vi "Gas_Release_Control.vi"(5 "Extra Commands":string, 6 "Density Ratio":string="Carrier 1 only", 7 "Strength (% by volume)":dbl format="%.3f", 8 "Stack flowrate (l/min)":dbl format="%.2f", 9 "Source Status":T2) -> (0 "error out":errorcluster, 1 "Flowrates (kg/min)":dbl[](array[numeric]) format="%.2f", 2 "Source Est Time (s)":dbl, 3 "Flowrates Achieved?":bool)   [LabVIEW 2011]
uses:
  ADAM Controls/Client_Source_Status.ctl
  ADAM Controls/Client_Source.ctl
  ADAM Controls/Channel_names.ctl
  ADAM Controls/Ch_description_ADAM.ctl
  ADAM Controls/Module_type_ADAM.ctl
  ADAM Controls/Function_ADAM.ctl
  ADAM Controls/Channel_State.ctl
  ADAM Controls/Calib_type_ADAM.ctl
  ADAM Controls/Address.ctl
  ADAM Controls/Update_scan_value.ctl
  Anemometry/Anemometry Sub Vis/Controls/In_Range.ctl
  Anemometry/Anemometry Sub Vis/Globals/Preference_global.vi
  Anemometry/Anemometry Sub Vis/Globals/Extra_Commands_Global.vi
panel:
  out "Error String":string
  out "Currently on":T1=enum."Get Source Clients"
  out "Status of other Clients":string[](array[string])
  out "Source already correct?":bool
  out "No Other Clients are Using Source?":bool
  out "Source Clients":string[](array[string])
  # "-Carrier 1 only\n-Carrier 2 only\n-Enter Ratio"
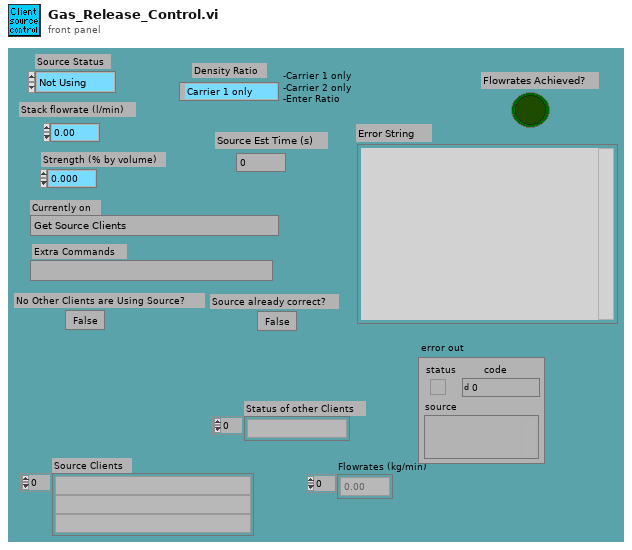
[diagram p1: front panel]
types:
  T1 = typedef "Client_Source.ctl" = enum16{"Start", "Get Source Clients", "Has this client liberty to control the source?", "Declare not using, other client already waiting", "Is the Source already correct?", "Declare waiting, other client is still using", "Control Hi-Tec", "Were the Hi-tecs able to achieve the flowrates?", "Declare source status", "Wait for source to Establish"}
  T2 = typedef "Client_Source_Status.ctl" = enum16{"Not Using", "Using", "Must Have"}
  T3 = typedef "Channel_names.ctl" = enum16{"Active Only", "Active + Off", "All Channels"}
  T4 = typedef "Ch_description_ADAM.ctl" = cluster{"Ch Name":string, "Type":T5, "Function":T6, "Ch State":T7, "Calibration type":T8, "A":dbl, "B":dbl, "C":dbl, "D":dbl, "Comments":string, "Address":T9, "String":string, "Duty":u16}
  T5 = typedef "Module_type_ADAM.ctl" = string
  T6 = typedef "Function_ADAM.ctl" = enum16{"Analogue Input", "Digital Input", "Event counter", "Event rate", "Analogue Output", "Digital Output", "Relay Output"}
  T7 = typedef "Channel_State.ctl" = enum16{"On", "Off", "Always On", "Always Off"}
  T8 = typedef "Calib_type_ADAM.ctl" = enum16{"Raw", "Bx + A", "Cx^2 + Bx + A", "Dx^3 + Cx^2 + Bx + A", "In Band", "Hi-Tec Q", "Hi-Tec M_dot", "Text"}
  T9 = typedef "Address.ctl" = cluster{"Main":i32, "Ch.":i32, "Sub":i32, "Port Name":string}
  T10 = typedef "Update_scan_value.ctl" = cluster{"Channel Name":string, "New Value":dbl}
  T11 = typedef "In_Range.ctl" = enum16{"%", "±", "% & ±"}
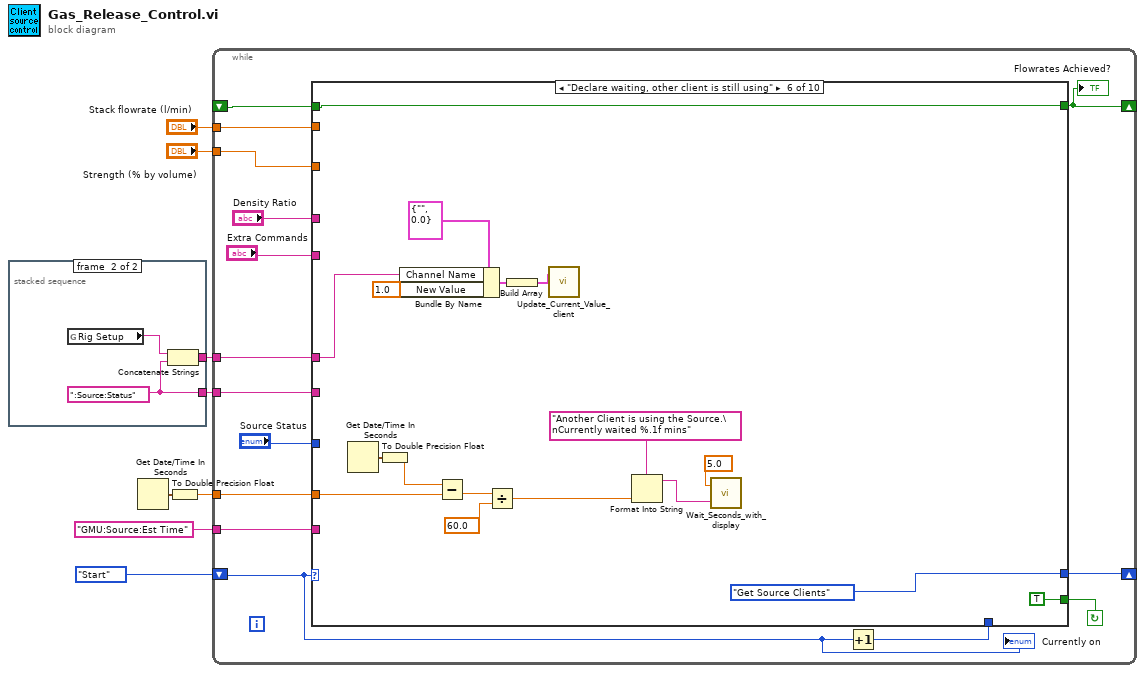
[diagram p0: block diagram]
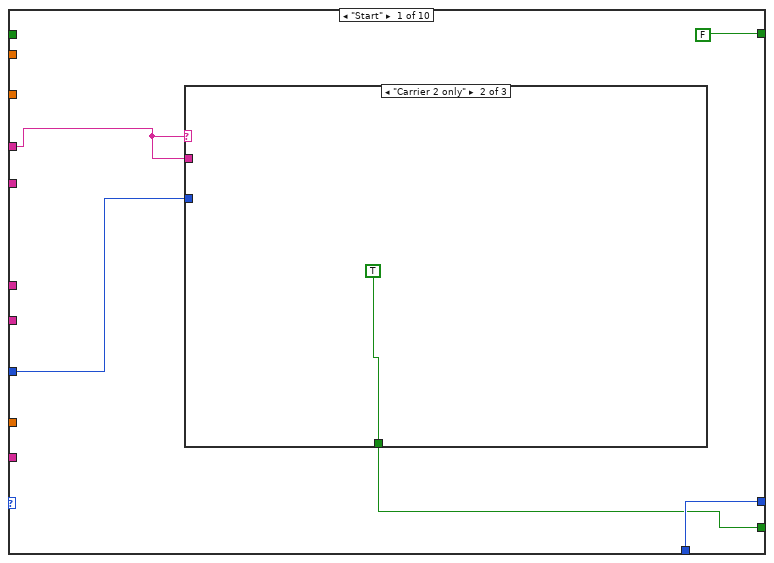
[diagram p2: hidden frame]
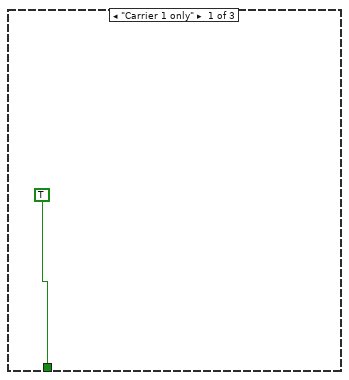
[diagram p3: hidden frame]
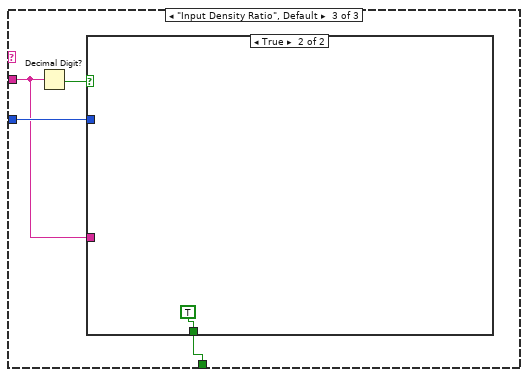
[diagram p4: hidden frame]
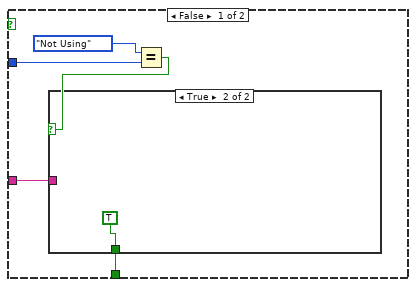
[diagram p5: hidden frame]
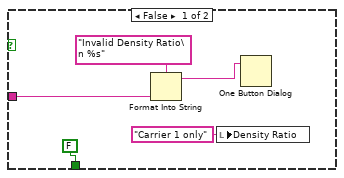
[diagram p6: hidden frame]
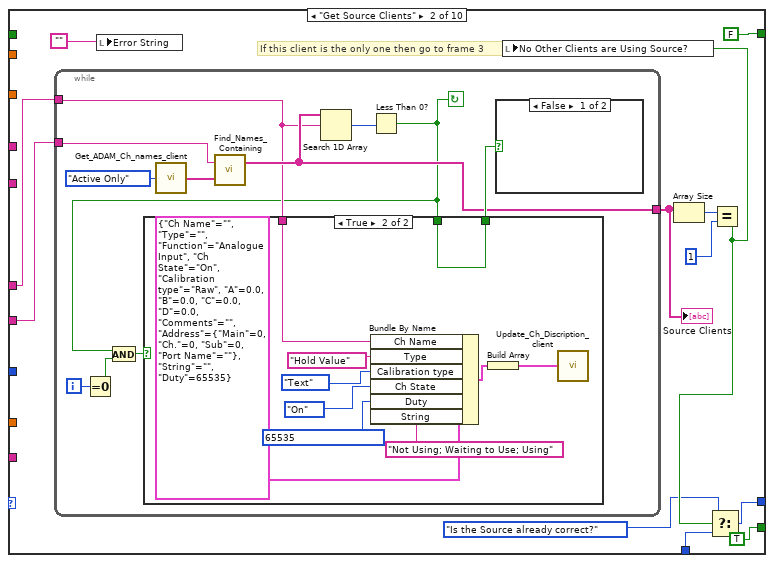
[diagram p7: hidden frame]
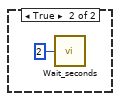
[diagram p8: hidden frame]
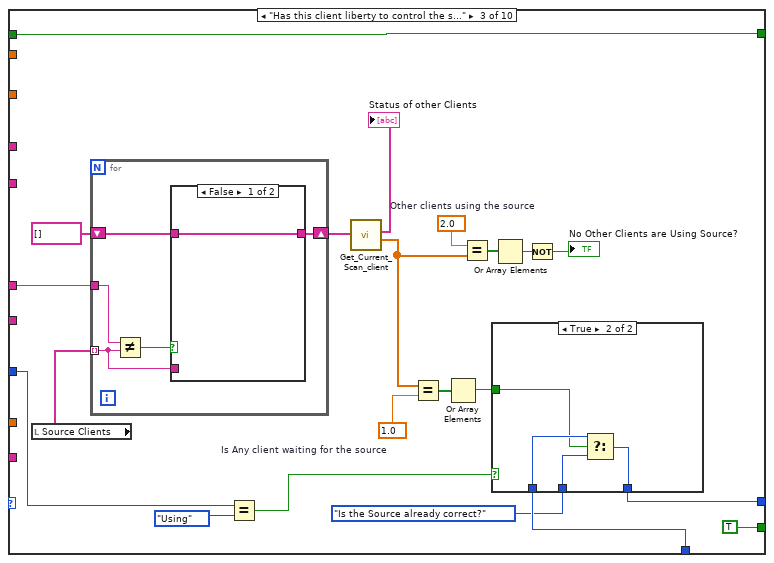
[diagram p10: hidden frame]
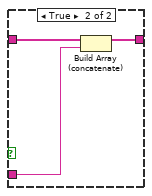
[diagram p12: hidden frame]
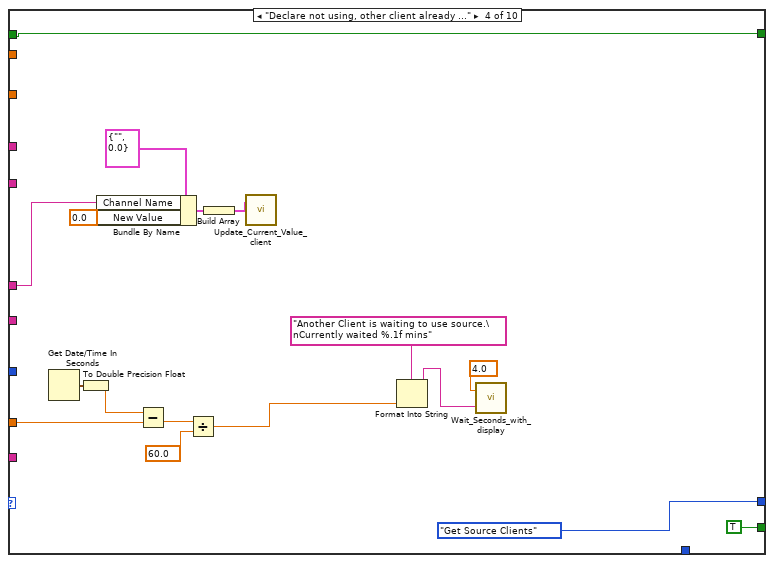
[diagram p13: hidden frame]
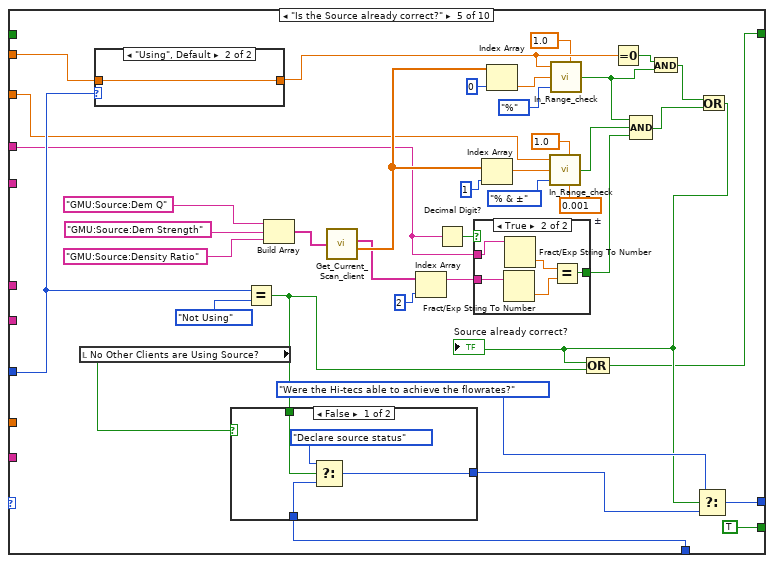
[diagram p14: hidden frame]
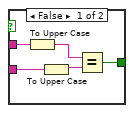
[diagram p15: hidden frame]
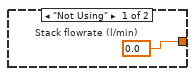
[diagram p16: hidden frame]
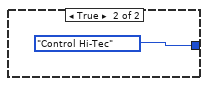
[diagram p17: hidden frame]
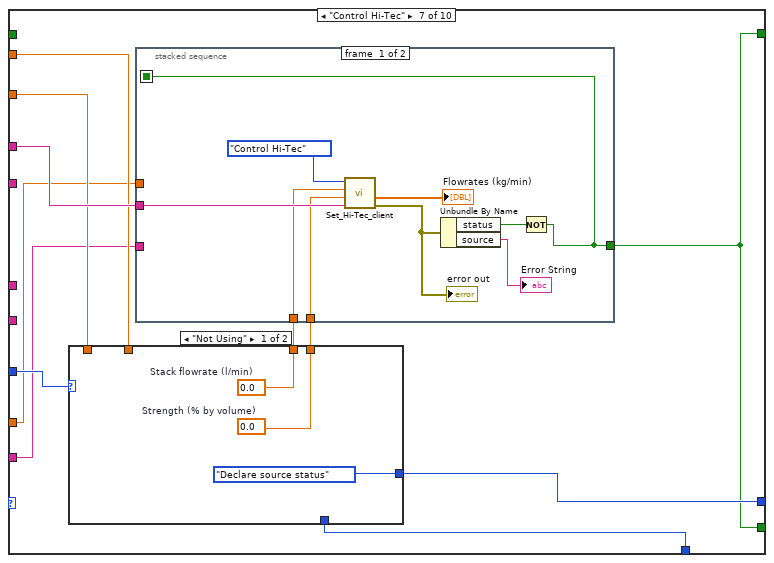
[diagram p18: hidden frame]
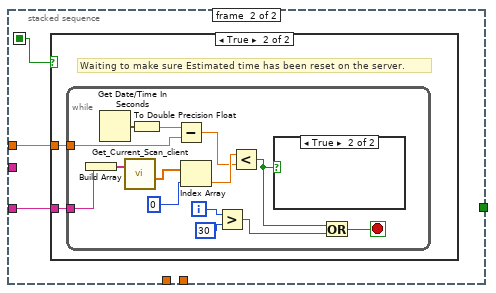
[diagram p19: hidden frame]
diagram:
  n1 = stacked-sequence {
    tunnel: [_ w11] -> w8
    tunnel: [_ w10] -> w7
    frame #0 {
      n2 = call "Run_EnFlo_Hub.vi"() -> ()  [unwired: 8 out]
    }
    frame #1 {
      w11 = ":Source:Status"
      n3 = global read "Preference_global.vi" "Rig Setup"() -> (w9:string)
      n4 = Concatenate Strings(w9, w11) -> (w10:string)
    }
  }
  n5 = Get Date/Time In Seconds() -> (seconds since 1Jan1904=w2:timestamp)
  n6 = To Double Precision Float(number=w2) -> (double precision float=w6:dbl)
  n7 = while {
    tunnel: w6 -> [w22]
    tunnel: w7 -> [w25]
    shift-left: Client_Source."Start" -> [w20]
    shift-right: [w21] -> _
    tunnel: w8 -> [w26]
    tunnel: "Stack flowrate (l/min)" -> [w16]
    tunnel: "Strength (% by volume)" -> [w15]
    shift-right: [w13] -> _
    shift-left: _ -> [w14]
    tunnel: "GMU:Source:Est Time" -> [w12]
    stop <- w24 continue-if-true
    n8 = Increment(x=w20) -> (x+1=w23:T1)
    n9 = case shown="\"Declare waiting, other client is still using\"" w20 {
      tunnel: w16 -> [_ _ _ _ w166 _ w217 w260 _ w308]
      tunnel: w15 -> [_ _ _ _ w147 _ w215 _ _ _]
      tunnel: "Density Ratio" -> [w30 _ _ _ w139 _ w220 _ _ _]
      tunnel: w26 -> [_ w61 _ _ _ _ _ _ _ _]
      tunnel: [w31 w57 w98 Client_Source."Get Source Clients" w175 Client_Source."Get Source Clients" w214 w262 w298 w314] -> w21
      tunnel: w25 -> [_ w60 w105 w131 _ w204 _ _ w304 _]
      tunnel: [w29 TRUE TRUE TRUE TRUE TRUE w210 TRUE TRUE FALSE] -> w24
      tunnel: w23 -> [w31 w56 w100 _ w167 _ w213 w261 w298 w314]
      tunnel: w22 -> [_ _ _ w129 _ w199 w211 _ _ _]
      tunnel: "Source Status" -> [w28 _ w89 _ w156 _ w219 w259 w302 w313]
      tunnel: "Extra Commands" -> [_ _ _ _ _ _ _ _ _ w311]
      tunnel: [FALSE FALSE w85 w121 w137 w194 w210 w258 w296 w309] -> w13
      tunnel: w14 -> [_ _ w85 w121 _ w194 _ _ w296 w309]
      tunnel: w12 -> [_ _ _ _ _ _ w212 w256 _ _]
      frame "Start" {
        n10 = case shown="\"Carrier 2 only\"" w30 {
          tunnel: w30 -> [_ _ w34]
          tunnel: [TRUE TRUE w35] -> w29
          tunnel: w28 -> [_ _ w36]
          frame "Carrier 1 only" {
            (unwired) TRUE
            (unwired) 0.0 ("Qc2")
          }
          frame "Carrier 2 only" {
            (unwired) TRUE
            (unwired) 0.0 ("Qc1")
          }
          frame "Input Density Ratio", Default {
            n11 = Decimal Digit?(1:w34) -> (0:w37:bool)
            n12 = case shown="True" w37 {
              tunnel: w36 -> [w41 _]
              tunnel: [w39 TRUE] -> w35
              tunnel: w34 -> [w38 _]
              frame False {
                n13 = Equal?(x=Client_Source_Status."Not Using" ("Source Status"), y=w41) -> (x = y?=w40:bool)
                n14 = case shown="True" w40 {
                  tunnel: [FALSE TRUE] -> w39
                  tunnel: w38 -> [w46 _]
                  frame False {
                    n15 = Format Into String(format string="Invalid Density Ratio\n %s", w46) -> (resulting string=w44:string)  [unwired: 2 in, 1 out]
                    n16 = local write "Density Ratio"("Carrier 1 only" ("Density Ratio")) -> ()
                    n17 = One Button Dialog(message=w44) -> ()  [unwired: 2 out]
                  }
                  frame True {
                  }
                }
              }
              frame True {
              }
            }
          }
        }
      }
      frame "Get Source Clients" {
        # "If this client is the only one then go to frame 3"
        n18 = while {
          tunnel: [w65] -> w54
          tunnel: w60 -> [w64]
          tunnel: w61 -> [w72]
          i -> [w69]
          stop <- w62 continue-if-true
          n19 = Equal To 0?(x=w69) -> (x = 0?=w68:bool)
          n20 = call "Get_ADAM_Ch_names_client.vi"("Channel names set"=Channel_names."Active Only") -> ("Ch names"=w70:string[])
          n21 = call "Find_Names_Containing.vi"("Ch names"=w70, "String to match"=w72) -> ("Matched Names"=w65:string[])  [unwired: 1 out]
          n22 = Search 1D Array(1D array=w65, element=w64) -> (index of element=w63:i32)  [unwired: 1 out]
          n23 = Less Than 0?(x=w63) -> (x < 0?=w62:bool)
          n24 = And(x=w62, y=w68) -> (x .and. y?=w67:bool)
          n25 = case shown="True" w67 {
            tunnel: w64 -> [_ w81]
            tunnel: [w74 w77] -> w66
            tunnel: w62 -> [w74 w77]
            frame False {
            }
            frame True {
              n26 = Bundle By Name(cluster=T4 {"Ch Name"="", "Type"="", "Function"=enum."Analogue Input", "Ch State"=enum."On", "Calibration type"=enum."Raw", "A"=0.0, "B"=0.0, "C"=0.0, "D"=0.0, "Comments"="", "Address"={"Main"=0, "Ch."=0, "Sub"=0, "Port Name"=""}, "String"="", "Duty"=65535} ("Ch Discription"), "Ch Name"=w81, "Type"=T5 "Hold Value", "Calibration type"=Calib_type_ADAM."Text", "Ch State"=Channel_State."On", "Duty"=u16 65535 ("Bundle Element"), "String"="Not Using; Waiting to Use; Using") -> (w79:T4)
              n27 = Build Array(w79) -> (w78:T4[])
              n28 = call "Update_Ch_Discription_client.vi"("Channels to update In"=w78) -> ()  [unwired: 1 out]
            }
          }
          n29 = case shown="False" w66 {
            frame False {
            }
            frame True {
              n30 = call "Wait_seconds.vi"("Seconds to wait"=u32 2) -> ()
            }
          }
        }
        "Source Clients" <- w54
        n31 = local write "Error String"("") -> ()
        n32 = Array Size(array=w54) -> (size(s)=w59:i32)
        n33 = Equal?(x=w59, y=1) -> (x = y?=w53:bool)
        n34 = local write "No Other Clients are Using Source?"(w53) -> ()
        n35 = Select(t=Client_Source."Is the Source already correct?", s=w53, f=w56) -> (s? t:f=w57:T1)
      }
      frame "Has this client liberty to control the source?" {
        w97 = 2.0  # Other clients using the source
        w103 = 1.0  # Is Any client waiting for the source
        n36 = local read "Source Clients"() -> (w99:string[])
        n37 = for {
          tunnel: w99 -> [w111] mode=indexing
          tunnel: w105 -> [w115]
          shift-right: [w112] -> w95
          shift-left: string[] [] -> [w113]
          n38 = Not Equal?(x=w115, y=w111) -> (x != y?=w114:bool)
          n39 = case shown="False" w114 {
            tunnel: w113 -> [w116 w119]
            tunnel: [w116 w118] -> w112
            tunnel: w111 -> [_ w117]
            frame False {
            }
            frame True {
              n40 = Build Array (concatenate)(w119, w117) -> (w118:string[])
            }
          }
        }
        n41 = Equal?(x=w89, y=Client_Source_Status."Using" ("Source Status")) -> (x = y?=w88:bool)
        n42 = call "Get_Current_Scan_client.vi"("ADAM Ch Names"=w95) -> ("String values"=→"Status of other Clients":string[], "Numerical Values"=w92:dbl[])  [unwired: 2 out]
        n43 = Equal?(x=w92, y=w103) -> (x = y?=w102:bool[])
        n44 = Or Array Elements(Boolean array=w102) -> (logical OR=w93:bool)
        n45 = Equal?(x=w97, y=w92) -> (x = y?=w96:bool[])
        n46 = case shown="True" w88 {
          tunnel: w100 -> [_ w110]
          tunnel: [w106 w109] -> w98
          tunnel: w93 -> [_ w108]
          tunnel: Client_Source."Is the Source already correct?" -> [w106 w107]
          frame False {
          }
          frame True {
            n47 = Select(t=w110, s=w108, f=w107) -> (s? t:f=w109:T1)
          }
        }
        n48 = Or Array Elements(Boolean array=w96) -> (logical OR=w91:bool)
        n49 = Not(x=w91) -> (.not. x?=→"No Other Clients are Using Source?":bool)
      }
      frame "Declare not using, other client already waiting" {
        n50 = Get Date/Time In Seconds() -> (seconds since 1Jan1904=w120:timestamp)
        n51 = To Double Precision Float(number=w120) -> (double precision float=w130:dbl)
        n52 = Bundle By Name(cluster=T10 {"Channel Name"="", "New Value"=0.0} ("Update Scan Value Cluster"), "Channel Name"=w131, "New Value"=0.0 ("Bundle Element")) -> (w134:T10)
        n53 = Subtract(x=w130, y=w129) -> (x-y=w128:dbl)
        n54 = Divide(x=w128, y=60.0) -> (x/y=w122:dbl)
        n55 = Build Array(w134) -> (w133:T10[])
        n56 = call "Update_Current_Value_client.vi"("Update array in"=w133) -> ()  [unwired: 1 in]
        n57 = Format Into String(format string="Another Client is waiting to use source.\nCurrently waited %.1f mins" ("Format String"), w122) -> (resulting string=w125:string)  [unwired: 2 in, 1 out]
        n58 = call "Wait_Seconds_with_display.vi"("Message"=w125, "Seconds to wait"=4.0) -> ()  [unwired: 2 out]
      }
      frame "Is the Source already correct?" {
        w144 = 0.001  # ±
        n59 = local read "No Other Clients are Using Source?"() -> (w169:bool)
        n60 = case shown="\"Using\", Default" w156 {
          tunnel: [w186 w187] -> w154
          tunnel: w166 -> [_ w187]
          frame "Not Using" {
            w186 = 0.0  # Stack flowrate (l/min)
          }
          frame "Using", Default {
          }
        }
        n61 = Equal?(x=w156, y=Client_Source_Status."Not Using" ("Source Status")) -> (x = y?=w155:bool)
        n62 = case shown="False" w169 {
          tunnel: [w191 Client_Source."Control Hi-Tec"] -> w168
          tunnel: w167 -> [w190 _]
          tunnel: w155 -> [w189 _]
          frame False {
            n63 = Select(t=Client_Source."Declare source status", s=w189, f=w190) -> (s? t:f=w191:T1)
          }
          frame True {
          }
        }
        n64 = Build Array("GMU:Source:Dem Q", "GMU:Source:Dem Strength", "GMU:Source:Density Ratio") -> (w171:string[])
        n65 = call "Get_Current_Scan_client.vi"("ADAM Ch Names"=w171) -> ("String values"=w141:string[], "Numerical Values"=w162:dbl[])  [unwired: 2 out]
        n66 = Index Array(array=w141, index=2 ("Index")) -> (element=w140:string)
        n67 = Decimal Digit?(1:w139) -> (0:w143:bool)
        n68 = case shown="True" w143 {
          tunnel: [w179 w182] -> w138
          tunnel: w139 -> [w178 w184]
          tunnel: w140 -> [w177 w185]
          frame False {
            n69 = To Upper Case(1:w178) -> (0:w180:string)
            n70 = To Upper Case(1:w177) -> (0:w176:string)
            n71 = Equal?(x=w180, y=w176) -> (x = y?=w179:bool)
          }
          frame True {
            n72 = Fract/Exp String To Number(string=w185) -> (number=w181:dbl)  [unwired: 4 out]
            n73 = Fract/Exp String To Number(string=w184) -> (number=w183:dbl)  [unwired: 4 out]
            n74 = Equal?(x=w183, y=w181) -> (x = y?=w182:bool)
          }
        }
        n75 = Index Array(array=w162, index=1 ("Index")) -> (element=w146:dbl)
        n76 = Index Array(array=w162, index=0 ("Index")) -> (element=w153:dbl)
        n77 = call "In_Range_check.vi"("±"=w144, "%"=1.0, "Mode"=In_Range."% & ±", "Value"=w146, "Setpoint"=w147) -> ("In Range"=w145:bool)  [unwired: 2 out]
        n78 = call "In_Range_check.vi"("%"=1.0, "Mode"=In_Range."%", "Value"=w153, "Setpoint"=w154) -> ("In Range"=w152:bool)  [unwired: 1 in, 2 out]
        n79 = Equal To 0?(x=w154) -> (x = 0?=w161:bool)
        n80 = Compound Arithmetic op=AND(w152, w145, w138) -> (w159:bool)
        n81 = And(x=w161, y=w152) -> (x .and. y?=w160:bool)
        n82 = Or(x=w160, y=w159) -> (x .or. y?=w158:bool)
        "Source already correct?" <- w158
        n83 = Compound Arithmetic op=OR(w158, w155) -> (w137:bool)
        n84 = Select(t=Client_Source."Were the Hi-tecs able to achieve the flowrates?", s=w158, f=w168) -> (s? t:f=w175:T1)
      }
      frame "Declare waiting, other client is still using" {
        n85 = Get Date/Time In Seconds() -> (seconds since 1Jan1904=w193:timestamp)
        n86 = To Double Precision Float(number=w193) -> (double precision float=w202:dbl)
        n87 = Bundle By Name(cluster=T10 {"Channel Name"="", "New Value"=0.0} ("Update Scan Value Cluster"), "Channel Name"=w204, "New Value"=1.0 ("Bundle Element")) -> (w207:T10)
        n88 = Subtract(x=w202, y=w199) -> (x-y=w201:dbl)
        n89 = Divide(x=w201, y=60.0) -> (x/y=w195:dbl)
        n90 = Build Array(w207) -> (w206:T10[])
        n91 = call "Update_Current_Value_client.vi"("Update array in"=w206) -> ()  [unwired: 1 in]
        n92 = Format Into String(format string="Another Client is using the Source.\nCurrently waited %.1f mins" ("Format String"), w195) -> (resulting string=w198:string)  [unwired: 2 in, 1 out]
        n93 = call "Wait_Seconds_with_display.vi"("Message"=w198, "Seconds to wait"=5.0) -> ()  [unwired: 2 out]
      }
      frame "Control Hi-Tec" {
        n94 = case shown="\"Not Using\"" w219 {
          tunnel: [w252 w255] -> w218
          tunnel: w217 -> [_ w255]
          tunnel: [w251 w254] -> w216
          tunnel: w215 -> [_ w254]
          tunnel: [Client_Source."Declare source status" w253] -> w214
          tunnel: w213 -> [_ w253]
          frame "Not Using" {
            w251 = 0.0  # Strength (% by volume)
            w252 = 0.0  # Stack flowrate (l/min)
          }
          frame "Using", Default {
          }
        }
        n95 = stacked-sequence {
          seq-local: [w221 _] -> [_ w230]
          tunnel: w220 -> [w228 _]
          tunnel: w218 -> [w226 _]
          tunnel: w216 -> [w225 _]
          tunnel: w212 -> [_ w232]
          tunnel: w211 -> [_ w231]
          tunnel: [w221 _] -> w210
          frame #0 {
            n96 = call "Set_Hi-Tec_client.vi"("Density Ratio"=w228, "Strength (% by volume)"=w225, "Stack flowrate (l/min)"=w226, "Mode"=enum16{"Control Hi-Tec", "Check Hi-Tec Demands"}."Control Hi-Tec") -> ("error out"=w224:errorcluster, "Flowrates (kg/min)"=→"Flowrates (kg/min)":dbl[])  [unwired: 1 in, 3 out]
            "error out" <- w224
            n97 = Unbundle By Name(w224) -> ("status"=w222:bool, "source"=→"Error String":string)
            n98 = Not(x=w222) -> (.not. x?=w221:bool)
          }
          frame #1 {
            n99 = case shown="True" w230 {
              tunnel: w232 -> [_ w234]
              tunnel: w231 -> [_ w233]
              frame False {
              }
              frame True {
                # "Waiting to make sure Estimated time has been reset on the server."
                n100 = while {
                  tunnel: w234 -> [w247]
                  tunnel: w233 -> [w242]
                  i -> [w239]
                  stop <- w235 stop-if-true
                  n101 = Build Array(w247) -> (w248:string[])
                  n102 = Get Date/Time In Seconds() -> (seconds since 1Jan1904=w244:timestamp)
                  n103 = call "Get_Current_Scan_client.vi"("ADAM Ch Names"=w248) -> ("Numerical Values"=w246:dbl[])  [unwired: 3 out]
                  n104 = To Double Precision Float(number=w244) -> (double precision float=w243:dbl)
                  n105 = Subtract(x=w243, y=w242) -> (x-y=w240:dbl)
                  n106 = Index Array(array=w246, index=0) -> (element=w241:dbl)
                  n107 = Greater?(x=w239, y=30) -> (0:w236:bool)
                  n108 = Less?(x=w241, y=w240) -> (x < y?=w237:bool)
                  n109 = case shown="True" w237 {
                    frame False {
                      n110 = Wait (ms)(milliseconds to wait=u32 1000) -> ()  [unwired: 1 out]
                    }
                    frame True {
                    }
                  }
                  n111 = Or(x=w237, y=w236) -> (x .or. y?=w235:bool)
                }
              }
            }
          }
        }
      }
      frame "Were the Hi-tecs able to achieve the flowrates?" {
        n112 = Get Date/Time In Seconds() -> (seconds since 1Jan1904=w257:timestamp)
        n113 = To Double Precision Float(number=w257) -> (double precision float=w264:dbl)
        n114 = while {
          tunnel: w259 -> [w272]
          tunnel: w260 -> [w270]
          tunnel: [w268] -> w263
          tunnel: w264 -> [w285]
          tunnel: [w268] -> w258
          tunnel: w256 -> [w266]
          stop <- w281 continue-if-true
          w269 = 0.1  # ±
          w277 = 1.0  # %
          n115 = case shown="\"Using\", Default" w272 {
            tunnel: [w290 w291] -> w271
            tunnel: w270 -> [_ w291]
            frame "Not Using" {
              w290 = 0.0  # Stack flowrate (l/min)
            }
            frame "Using", Default {
            }
          }
          n116 = Get Date/Time In Seconds() -> (seconds since 1Jan1904=w267:timestamp)
          n117 = To Double Precision Float(number=w267) -> (double precision float=w286:dbl)
          n118 = Subtract(x=w286, y=w285) -> (x-y=w284:dbl)
          n119 = Build Array("GMU:Source:Dem Q", w266) -> (w289:string[])
          n120 = Less?(x=w284, y=120.0) -> (x < y?=w282:bool)
          n121 = call "Get_Current_Scan_client.vi"("ADAM Ch Names"=w289) -> ("Numerical Values"=w275:dbl[])  [unwired: 3 out]
          n122 = Index Array(array=w275, index=1 ("Index")) -> (element=w287:dbl)
          "Source Est Time (s)" <- w287
          n123 = Index Array(array=w275, index=0 ("Index")) -> (element=w279:dbl)
          n124 = Greater Than 0?(x=w287) -> (x > 0?=w273:bool)
          n125 = call "In_Range_check.vi"("±"=w269, "%"=w277, "Mode"=In_Range."% & ±", "Value"=w279, "Setpoint"=w271) -> ("In Range"=w274:bool)  [unwired: 2 out]
          n126 = And(x=w274, y=w273) -> (x .and. y?=w268:bool)
          n127 = Compound Arithmetic op=AND(invert w268, w282) -> (w281:bool)
          n128 = case shown="True" w281 {
            frame False {
            }
            frame True {
              n129 = Wait (ms)(milliseconds to wait=u32 1000) -> ()  [unwired: 1 out]
            }
          }
        }
        n130 = case shown="True" w263 {
          tunnel: [Client_Source."Control Hi-Tec" w295] -> w262
          tunnel: w261 -> [_ w295]
          frame False {
            n131 = local write "Source Status"(Client_Source_Status."Not Using" ("Source Status")) -> ()
          }
          frame True {
          }
        }
      }
      frame "Declare source status" {
        n132 = case shown="\"Not Using\"" w302 {
          tunnel: [0.0 2.0 2.0] -> w297
          frame "Not Using" {
          }
          frame "Using" {
          }
          frame "Must Have" {
          }
        }
        n133 = Bundle By Name(cluster=T10 {"Channel Name"="", "New Value"=0.0} ("Update Scan Value Cluster"), "Channel Name"=w304, "New Value"=w297) -> (w300:T10)
        n134 = Build Array(w300) -> (w299:T10[])
        n135 = call "Update_Current_Value_client.vi"("Update array in"=w299) -> ()  [unwired: 1 in]
      }
      frame "Wait for source to Establish" {
        n136 = Not Equal?(x=Client_Source_Status."Not Using" ("Source Status"), y=w313) -> (x != y?=w310:bool)
        n137 = case shown="True" w310 {
          tunnel: w311 -> [_ w332]
          tunnel: w308 -> [_ w321]
          frame False {
          }
          frame True {
            n138 = global read "Extra_Commands_Global.vi" "Establish Exp Conditions (s)"() -> (w333:string)
            n139 = global read "Preference_global.vi" "Default Source Establishment Time (s)"() -> (w324:dbl)
            n140 = Equal To 0?(x=w321) -> (x = 0?=w319:bool)
            n141 = Divide(x=100.0, y=w321) -> (x/y=w318:dbl)
            n142 = local read "Source Est Time (s)"() -> (w325:dbl)
            n143 = Not A Number/Path/Refnum?(number/path/refnum=w325) -> (NaN/Path/Refnum?=w329:bool)
            n144 = call "Extra_Commands.vi"("String to Search"=w332, "Command"=w333) -> ("Numeric Value"=w326:dbl, "Command Found"=w327:bool)  [unwired: 1 in, 3 out]
            n145 = Select(t=w326, s=w327, f=w324) -> (s? t:f=w323:dbl)
            n146 = Select(t=0.0, s=w319, f=w318) -> (s? t:f=w316:dbl)
            n147 = Add(x=w316, y=w323) -> (x+y=w322:dbl)
            n148 = Subtract(x=w322, y=w325) -> (x-y=w328:dbl)
            n149 = Greater Than 0?(x=w328) -> (x > 0?=w331:bool)
            n150 = Or(x=w331, y=w329) -> (x .or. y?=w330:bool)
            n151 = case shown="True" w330 {
              tunnel: w329 -> [_ w337]
              tunnel: w322 -> [_ w336]
              tunnel: w328 -> [_ w335]
              frame False {
              }
              frame True {
                n152 = Select(t=w336, s=w337, f=w335) -> (s? t:f=w334:dbl)
                n153 = call "Wait_Seconds_with_display.vi"("Message"="Establishing Source", "Seconds to wait"=w334) -> ()  [unwired: 2 out]
              }
            }
          }
        }
      }
    }
    "Flowrates Achieved?" <- w13
    "Currently on" <- w20
  }
